vi "MMI_ButtonSkin_StrDismantle.vi"(1 "LogEvent":refnum<vi>, 2 "VCI_CAN_OBJ_R":T1) -> (0 "MMI_ButtonSkin_CmdCluster":T2 {"SVA声音报警设置" items=["无请求", "禁止", "启用"]; "IPK-HUD-MMI皮肤联动" items=["联动", "未联动"]; "总里程清零命令" items=["无命令", "清零"]; "指示目的地距离单位" items=["无显示", "Meter", "KiloMeter"]; "MMI激活HUD" items=["无", "未激活", "已激活"]; "皮肤模式" items=["皮肤1", "皮肤2", "皮肤3"]; "方向盘多功能开关模式" items=["MMImode", "IPKmode", "HUDmode"]; "方向盘返回键动作" items=["未按下", "短按", "长按", "长按不松手"]; "方向盘确认键动作" items=["未按下", "短按", "长按", "长按不松手"]; "方向盘下指示键动作" items=["未按下", "短按", "长按", "长按不松手"]; "方向盘上指示键动作" items=["未按下", "短按", "长按", "长按不松手"]; "方向盘左指示键动作" items=["未按下", "短按", "长按", "长按不松手"]; "方向盘右指示键动作" items=["未按下", "短按", "长按", "长按不松手"]})   [LabVIEW 2013]
uses:
  Log.ctl
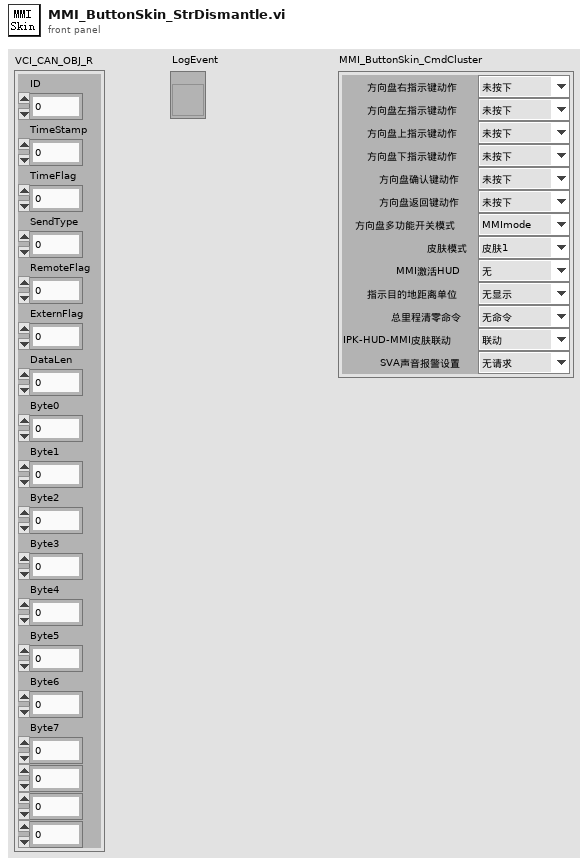
[diagram p1: front panel]
types:
  T1 = cluster{"ID":u32, "TimeStamp":u32, "TimeFlag":u8, "SendType":u8, "RemoteFlag":u8, "ExternFlag":u8, "DataLen":u8, "Byte0":u8, "Byte1":u8, "Byte2":u8, "Byte3":u8, "Byte4":u8, "Byte5":u8, "Byte6":u8, "Byte7":u8, u8, u8, u8}
  T2 = cluster{"方向盘右指示键动作":u16, "方向盘左指示键动作":u16, "方向盘上指示键动作":u16, "方向盘下指示键动作":u16, "方向盘确认键动作":u16, "方向盘返回键动作":u16, "方向盘多功能开关模式":u16, "皮肤模式":u16, "MMI激活HUD":u16, "指示目的地距离单位":u16, "总里程清零命令":u16, "IPK-HUD-MMI皮肤联动":u16, "SVA声音报警设置":u16}
  T3 = typedef "Log.ctl" = cluster{"Event":string, "Value":variant}
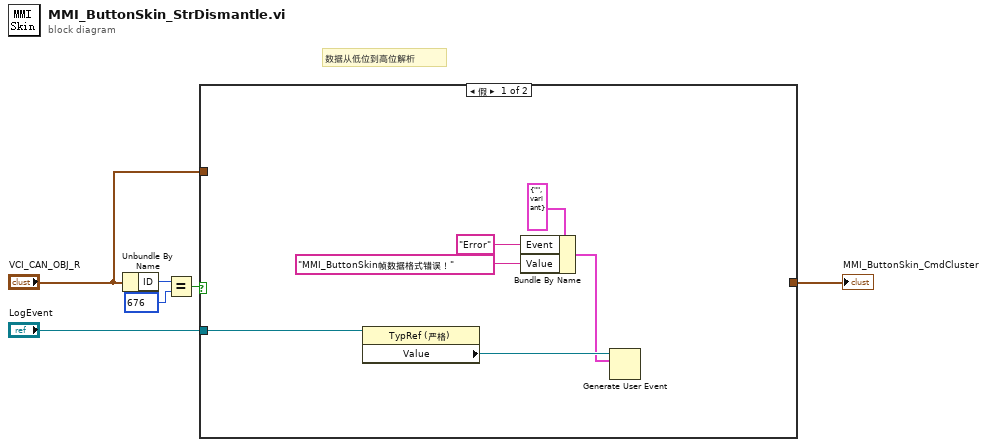
[diagram p0: block diagram]
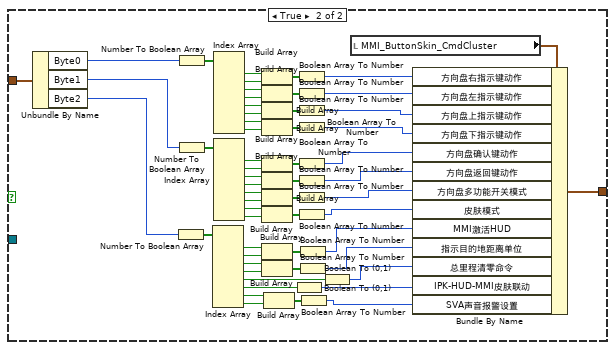
[diagram p2: hidden frame]
diagram:
  # "数据从低位到高位解析"
  n1 = Unbundle By Name("VCI_CAN_OBJ_R") -> ("ID"=w5:u32)
  n2 = Equal?(x=w5, y=u16 676) -> (x = y?=w3:bool)
  n3 = case shown="假" w3 {
    tunnel: [_ w17] -> w6
    tunnel: "VCI_CAN_OBJ_R" -> [_ w16]
    tunnel: "LogEvent" -> [w8 _]
    frame False {
      n4 = property class="TypRef (严格)"(reference=w8) -> ("Value"=w12:refnum<user-event>)  [unwired: 1 in, 2 out]
      n5 = Bundle By Name(cluster=T3 {"Event"="", "Value"=variant} ("Log"), "Event"="Error", "Value"="MMI_ButtonSkin帧数据格式错误！" ("消息")) -> (w9:T3)
      n6 = Generate User Event(user event=w12, event data cluster=w9) -> ()  [unwired: 2 in, 2 out]
    }
    frame True {
      n7 = Unbundle By Name(w16) -> ("Byte0"=w15:u8, "Byte1"=w14:u8, "Byte2"=w13:u8)
      n8 = Number To Boolean Array(number=w13) -> (Boolean array=w34:bool[])
      n9 = Number To Boolean Array(number=w15) -> (Boolean array=w68:bool[])
      n10 = Number To Boolean Array(number=w14) -> (Boolean array=w39:bool[])
      n11 = Index Array(array=w34) -> (element #1=w32:bool, element #2=w31:bool, element #3=w28:bool, element #4=w27:bool, element #5=w25:bool, element #6=w23:bool, element #7=w20:bool, element #8=w19:bool)  [unwired: 8 in]
      n12 = Index Array(array=w68) -> (element #1=w66:bool, element #2=w65:bool, element #3=w62:bool, element #4=w61:bool, element #5=w58:bool, element #6=w57:bool, element #7=w55:bool, element #8=w53:bool)  [unwired: 8 in]
      n13 = Index Array(array=w39) -> (element #1=w41:bool, element #2=w42:bool, element #3=w44:bool, element #4=w45:bool, element #5=w47:bool, element #6=w48:bool, element #7=w49:bool, element #8=w51:bool)  [unwired: 8 in]
      n14 = Build Array(w66, w65) -> (w67:bool[])
      n15 = Build Array(w62, w61) -> (w63:bool[])
      n16 = Build Array(w58, w57) -> (w59:bool[])
      n17 = Build Array(w55, w53) -> (w54:bool[])
      n18 = Build Array(w41, w42) -> (w40:bool[])
      n19 = Build Array(w44, w45) -> (w43:bool[])
      n20 = Build Array(w47, w48) -> (w46:bool[])
      n21 = Build Array(w49, w51) -> (w50:bool[])
      n22 = Build Array(w32, w31) -> (w33:bool[])
      n23 = Build Array(w28, w27) -> (w29:bool[])
      n24 = Build Array(w20, w19) -> (w21:bool[])
      n25 = Boolean To (0,1)(Boolean=w23) -> (0, 1=w22:i16)
      n26 = Boolean Array To Number(Boolean array=w67) -> (number=w64:u32)
      n27 = Boolean Array To Number(Boolean array=w63) -> (number=w60:u32)
      n28 = Boolean Array To Number(Boolean array=w59) -> (number=w56:u32)
      n29 = Boolean Array To Number(Boolean array=w54) -> (number=w52:u32)
      n30 = Boolean Array To Number(Boolean array=w40) -> (number=w38:u32)
      n31 = Boolean Array To Number(Boolean array=w43) -> (number=w37:u32)
      n32 = Boolean Array To Number(Boolean array=w46) -> (number=w36:u32)
      n33 = Boolean Array To Number(Boolean array=w50) -> (number=w35:u32)
      n34 = Boolean Array To Number(Boolean array=w33) -> (number=w30:u32)
      n35 = Boolean Array To Number(Boolean array=w29) -> (number=w26:u32)
      n36 = Boolean Array To Number(Boolean array=w21) -> (number=w18:u32)
      n37 = Boolean To (0,1)(Boolean=w25) -> (0, 1=w24:i16)
      n38 = local read "MMI_ButtonSkin_CmdCluster"() -> (w69:T2)
      n39 = Bundle By Name(cluster=w69, "方向盘右指示键动作"=w64, "方向盘左指示键动作"=w60, "方向盘上指示键动作"=w56, "方向盘下指示键动作"=w52, "方向盘确认键动作"=w38, "方向盘返回键动作"=w37, "方向盘多功能开关模式"=w36, "皮肤模式"=w35, "MMI激活HUD"=w30, "指示目的地距离单位"=w26, "总里程清零命令"=w24, "IPK-HUD-MMI皮肤联动"=w22, "SVA声音报警设置"=w18) -> (w17:T2)
    }
  }
  "MMI_ButtonSkin_CmdCluster" <- w6
